vi "Initialize HW.vi"(8 "error in (no error)":errorcluster, 11 "Switch in":refnum<class "Switch.lvclass">) -> (0 "error out":errorcluster, 3 "Switch out":refnum<class "Switch.lvclass">)   [LabVIEW 2020, in "Switch.lvclass"]
uses:
  Switch.lvclass
  Actuator.lvclass
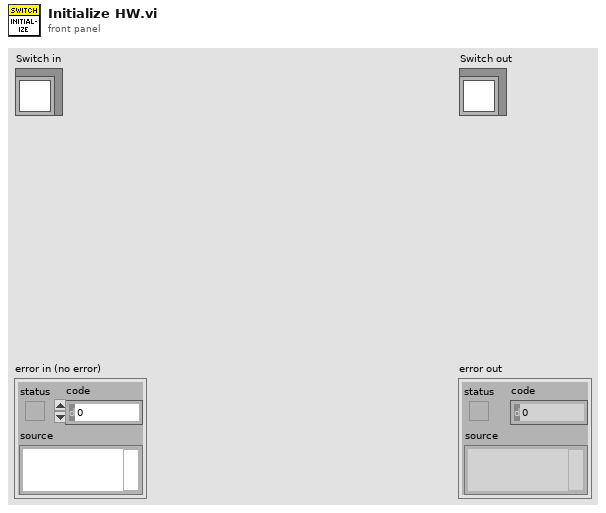
[diagram p1: front panel]
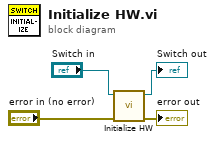
[diagram p0: block diagram]
diagram:
  n1 = call-parent "Initialize HW.vi"("error in (no error)"="error in (no error)", "Actuator in"="Switch in") -> ("error out"=→"error out":errorcluster, "Actuator out"=→"Switch out":refnum<class "Switch.lvclass">)  [unwired: 8 in]
